vi "SoundPlay15m.vi"   [LabVIEW 2014]
uses:
  isPlaying.vi
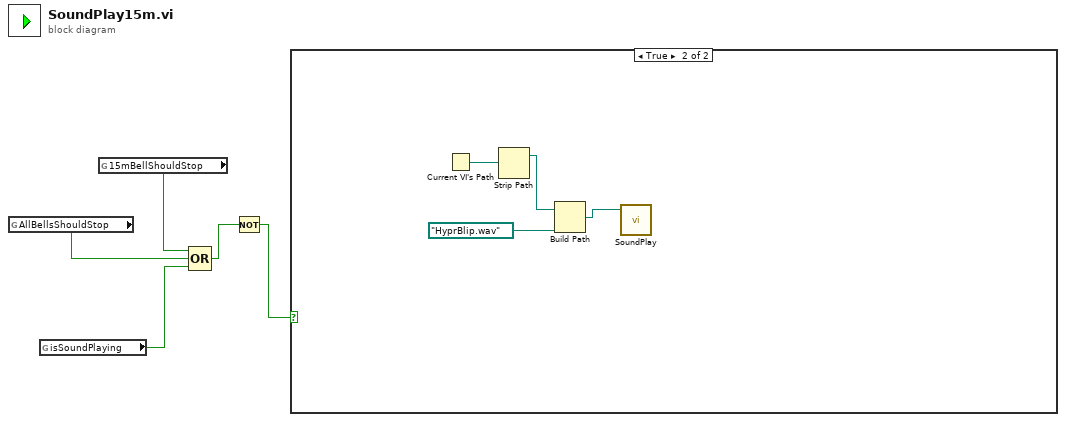
[diagram p0: block diagram]
diagram:
  n1 = global read "isPlaying.vi" "AllBellsShouldStop"() -> (w4:bool)
  n2 = global read "isPlaying.vi" "isSoundPlaying"() -> (w1:bool)
  n3 = global read "isPlaying.vi" "15mBellShouldStop"() -> (w5:bool)
  n4 = Compound Arithmetic op=OR(w5, w4, w1) -> (w3:bool)
  n5 = Not(x=w3) -> (.not. x?=w2:bool)
  n6 = case shown="True" w2 {
    frame False {
    }
    frame True {
      n7 = Current VI's Path() -> (path=w7:path)
      n8 = Strip Path(path=w7) -> (stripped path=w6:path)  [unwired: 1 out]
      n9 = Build Path(base path=w6, name or relative path=path "HyprBlip.wav") -> (appended path=w9:path)
      n10 = call "SoundPlay.vi"("Path to Sound file"=w9) -> ()  [unwired: 2 in, 1 out]
    }
  }
